vi "Read Template Path.vi"(8 "error in (no error)":errorcluster, 11 "CS++MessageMakerMain in":refnum<class "CS++MessageMakerMain.lvclass">) -> (0 "error out":errorcluster, 2 "Template Path":path, 3 "CS++MessageMakerMain out":refnum<class "CS++MessageMakerMain.lvclass">)   [LabVIEW 2014, in "CS++MessageMakerMain.lvlib" / "CS++MessageMakerMain.lvclass"]
uses:
  CS++MessageMakerMain.lvclass
  CS++MessageMakerMain.lvclass/CS++MessageMakerMain.ctl
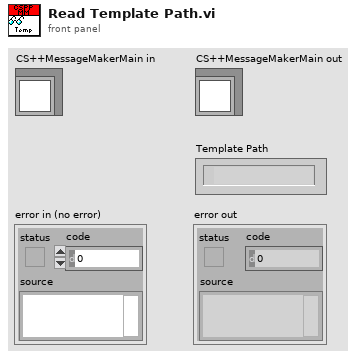
[diagram p1: front panel]
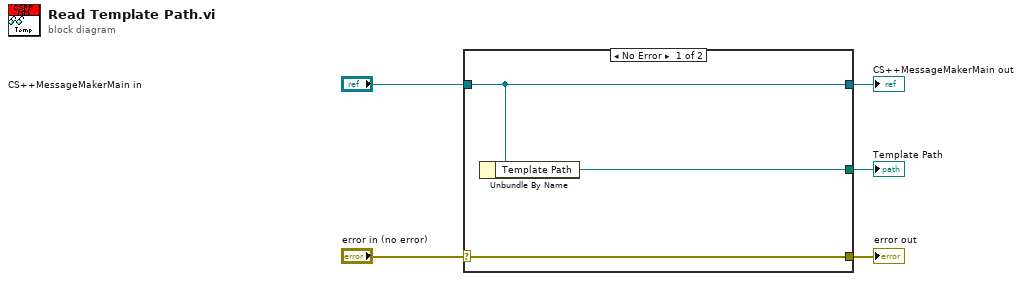
[diagram p0: block diagram]
diagram:
  n1 = case shown="No Error" "error in (no error)" {
    selector: "error in (no error)" -> [w8 w9]
    tunnel: [w8 w9] -> w4
    tunnel: [w7 w10] -> w2
    tunnel: "CS++MessageMakerMain in" -> [w7 w10]
    tunnel: [w6 _] -> w1
    frame No Error {
      n2 = Unbundle By Name(w7) -> ("Template Path"=w6:path)
    }
    frame Error {
    }
  }
  "error out" <- w4
  "CS++MessageMakerMain out" <- w2
  "Template Path" <- w1
